vi "Load Parameterized Executive.vi"(5 "Path Builder":refnum<class "IPath Builder.lvclass">, 6 "Folder":path, 7 "Compatibility Helper":refnum<class "ICompatibility Helper.lvclass">, 8 "error in (no error)":errorcluster, 9 "Persistence in":refnum<class "IPersist.lvclass">, 10 "Test Executive":refnum<class "ITest Executive.lvclass">, 11 "Test Executive Ref":refnum<data-value>) -> (0 "error out":errorcluster, 3 "Test Executive Ref out":refnum<data-value>)   [LabVIEW 2017, in "Test Executive.lvlib" / "TestExecutive Ref.lvclass"]
uses:
  <vilib>/gpm_packages/@cs/test-executive/Source/Test Executive/TestExecutive Ref/TestExecutive Ref.lvclass
  <vilib>/gpm_packages/@cs/test-executive/Source/Test Executive/ITestExecutive/ITest Executive.lvclass
  <vilib>/gpm_packages/@cs/persistence/source/IPersist/IPersist.lvclass
  <vilib>/gpm_packages/@cs/test-executive/Source/Path Builder/IPath Builder/IPath Builder.lvclass
  <vilib>/gpm_packages/@cs/test-executive/Source/Compatibility Helper/ICompatibility Helper.lvclass
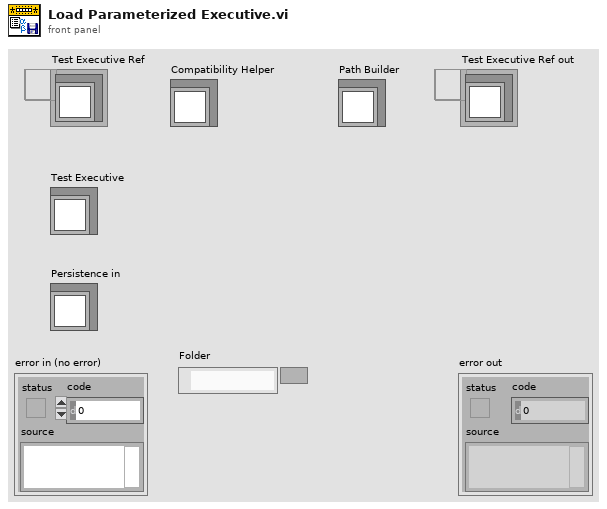
[diagram p1: front panel]
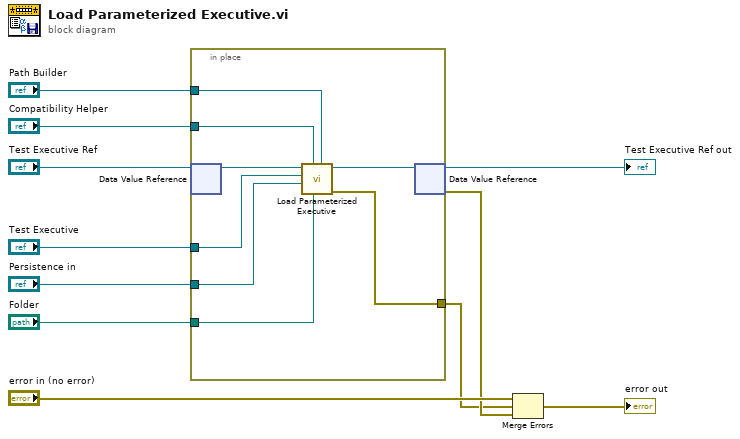
[diagram p0: block diagram]
diagram:
  n1 = in-place {
    in-place-border: "Test Executive" -> [w17]
    in-place-border: "Persistence in" -> [w16]
    in-place-border: "Folder" -> [w15]
    in-place-border: [w14] -> w3
    in-place-border: "Compatibility Helper" -> [w13]
    in-place-border: "Path Builder" -> [w12]
    n2 = in-place-dvr #1("Test Executive Ref") -> (w19:refnum<class "ITest Executive.lvclass">)  [unwired: 1 out]
    n3 = call-dynamic "Load Parameterized Executive.vi"("Path Builder"=w12, "Folder"=w15, "Compatibility Helper"=w13, "Persistence in"=w16, "Test Executive"=w17, "ITest Executive in"=w19) -> ("error out"=w14:errorcluster, "ITest Executive out"=w18:refnum<class "ITest Executive.lvclass">)  [unwired: 4 in]
    n4 = in-place-dvr #1(w18) -> (→"Test Executive Ref out":refnum<data-value>, w9:errorcluster)
  }
  n5 = Merge Errors("error in (no error)", w3, w9) -> (→"error out":errorcluster)
